vi "Stop Everything FGV.vi"(8 "error in (no error)":errorcluster, 11 "Stop Everything?":bool) -> (0 "error out":errorcluster, 3 "Stop?":bool)   [LabVIEW 2011]
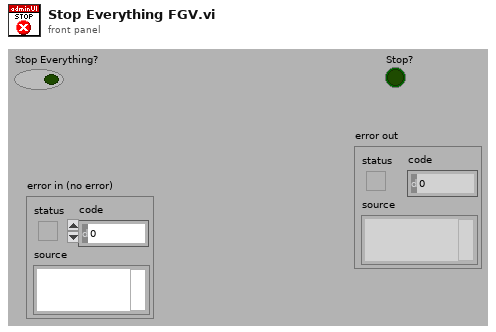
[diagram p1: front panel]
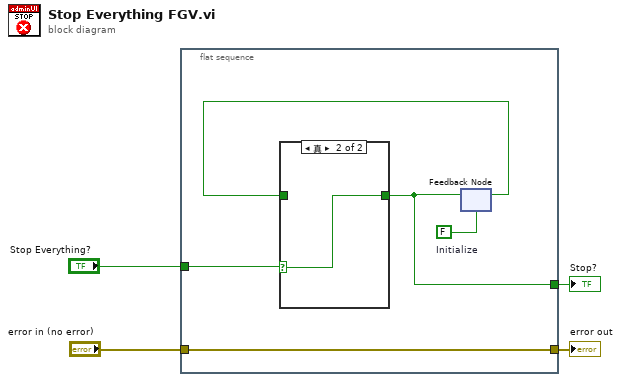
[diagram p0: block diagram]
diagram:
  n1 = flat-sequence {
    tunnel: "Stop Everything?" -> [w7]
    tunnel: [w6] -> w3
    tunnel: [w5] -> w1
    tunnel: "error in (no error)" -> [w5]
    frame #0 {
      w8 = FALSE  # Initialize
      n2 = feedback #1(w8) -> (w9:bool)
      n3 = case shown="真" w7 {
        selector: w7 -> [_ w11]
        tunnel: [w10 w11] -> w6
        tunnel: w9 -> [w10 _]
        frame False {
        }
        frame True {
        }
      }
      n4 = feedback-in #1(w6) -> ()
    }
  }
  "Stop?" <- w3
  "error out" <- w1
